vi "Change Samps_Cycle.vi"(0 "nCRD in":refnum<class "nCRD.lvclass">, 5 "error in":errorcluster) -> (14 "nCRD out":refnum<class "nCRD.lvclass">, 19 "error out":errorcluster)   [LabVIEW 2015, in "nCRD.lvclass"]
uses:
  nCRD.lvclass
  Session/Raw FPGA/FPGA Session.lvclass
  nCRD.lvclass/nCRD.ctl
  Session/Raw FPGA/FPGA Session.lvclass/FPGA Session.ctl
  Session/Raw FPGA/Read FPGA Ref.vi
  <vilib>/Utility/error.llb/Error Cluster From Error Code.vi
  <vilib>/rvi/errors/niLvFpgaAdjustHostInterfaceError.vi
  FPGA Ref.ctl
  <vilib>/rvi/interface/nirviReadWriteControl/nirviReadWriteControl.xnode
  FPGA Bitfiles/NickIO.lvbitx
  NiFpgaLv.dll
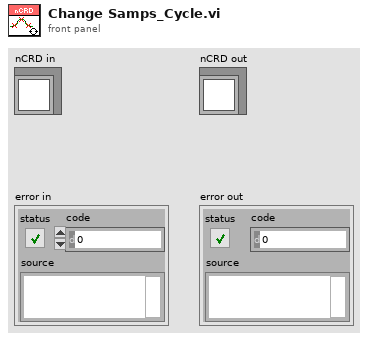
[diagram p1: front panel]
types:
  T1 = typedef "Session - Root.lvclass/Session Handle.ctl" = refnum<data-value>
  T2 = typedef "FPGA Ref.ctl" = refnum<k20>
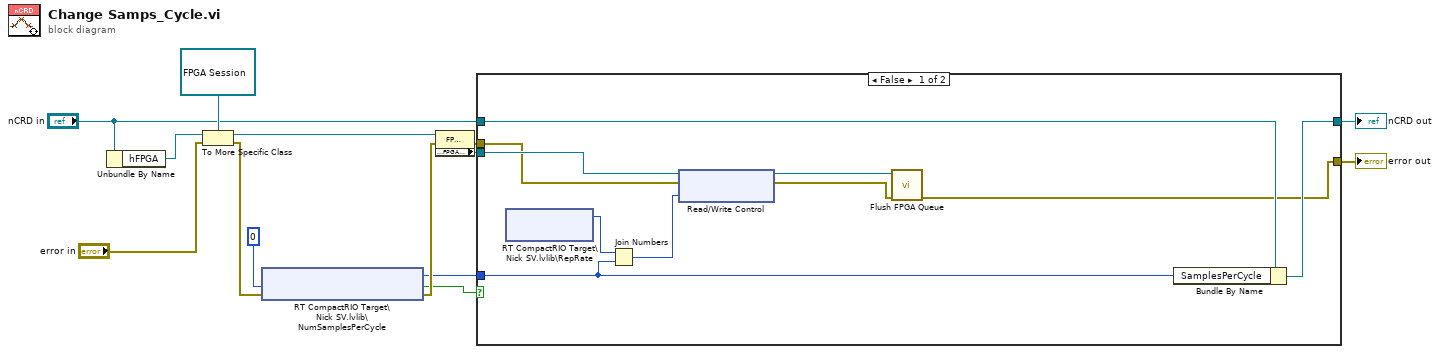
[diagram p0: block diagram]
diagram:
  n1 = Unbundle By Name("nCRD in") -> ("hFPGA"=w7:T1)
  n2 = To More Specific Class(target class=refnum<data-value> refnum ("hFPGA"), reference=w7, error in="error in") -> (specific class reference=w9:refnum<data-value>, error out=w12:errorcluster)
  n3 = shared-variable "RT CompactRIO Target\\Nick SV.lvlib\\NumSamplesPerCycle"(error in=w12, 0 ("ms timeout (0)")) -> (w1:u16, error out=w13:errorcluster, w2:bool)
  n4 = property class="FPGA Session"(reference=w9, error in=w13) -> (error out=w14:errorcluster, "Accessors:FPGA Ref"=w10:T2)  [unwired: 1 out]
  n5 = case shown="False" w2 {
    tunnel: [w24 w26] -> w5
    tunnel: "nCRD in" -> [w23 w26]
    tunnel: w10 -> [w21 _]
    tunnel: w1 -> [w17 _]
    tunnel: [w22 w25] -> w3
    tunnel: w14 -> [w19 w25]
    frame False {
      n6 = shared-variable "RT CompactRIO Target\\Nick SV.lvlib\\RepRate"() -> (w16:u16)  [unwired: 2 in, 2 out]
      n7 = Join Numbers(hi=w16, lo=w17) -> ((hi.lo)=w15:u32)
      n8 = xnode "Read/Write Control"("FPGA VI Reference In"=w21, "error in"=w19, "CRDSampData"=w15) -> ("FPGA VI Reference Out"=w20:T2, "error out"=w18:errorcluster)
      n9 = call "Flush FPGA Queue.vi"("error in (no error)"=w18, "Refnum in"=w20) -> ("error out"=w22:errorcluster)  [unwired: 9 in]
      n10 = Bundle By Name(cluster=w23, "SamplesPerCycle"=w17) -> (w24:refnum<class "nCRD.lvclass">)
    }
    frame True {
    }
  }
  "nCRD out" <- w5
  "error out" <- w3
